vi "PR Set Pulse.vi"(1 "PulseIndex":i32) -> (0 "function return":bool)   [LabVIEW 2022 SP3, in "BS6006PRPLUS.lvlib"]
doc: "The function sets the level of pulser of Pulser/Receiver. When the pulse repetition frequency is set to be higher than 5 kHz, the PulseIndex should be less than 12.\n\nextern \"C\" BS6006PRPLUS_API bool __cdecl PR_SetPulse(int PulseIndex);"
uses:
  BS6006PRPLUS.lvlib
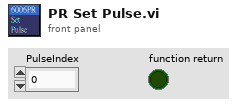
[diagram p1: front panel]
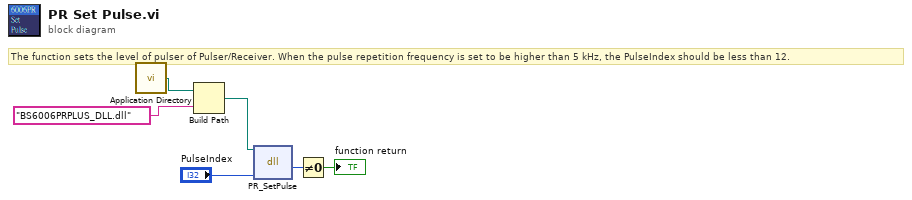
[diagram p0: block diagram]
diagram:
  # "The function sets the level of pulser of Pulser/Receiver. When the pulse repetition frequency is set to be higher than 5 kHz, the PulseIndex should be less than 12."
  n1 = call <vilib>:"Application Directory.vi"() -> ("Application Directory"=w3:path)
  n2 = Build Path(base path=w3, name or relative path="BS6006PRPLUS_DLL.dll") -> (appended path=w1:path)
  n3 = dll-call lib="E:/Broadsound_Program/PulserReceiver/6006PR PLUS/API/DLL/LabVIEW 15/VIs/BS6006PRPLUS_DLL.dll" fn="PR_SetPulse"(path in=w1, "PulseIndex"="PulseIndex") -> ("return type"=w5:u8)  [unwired: 3 in, 2 out]
  n4 = Not Equal To 0?(x=w5) -> (x != 0?=→"function return":bool)
